vi "Create Pattern Script(Special Frames).vi"(7 "Special Frame Type":T1, 8 "error in (no error)":errorcluster, 10 "Num of Timeset":u32, 11 "BML Pattern Creater in":refnum<class "BML Pattern Creater.lvclass">) -> (0 "error out":errorcluster, 2 "string out":string, 3 "BML Pattern Creater out":refnum<class "BML Pattern Creater.lvclass">)   [LabVIEW 2018, in "BML Pattern Creater.lvlib" / "BML Pattern Creater.lvclass"]
uses:
  BML Pattern Creater.lvclass
  Special Frame.ctl
  Interfaces/Protocol Interface.lvlibp/Interfaces/Protocol Interface/Pin State.ctl
  Interfaces/Protocol Interface.lvlibp/Interfaces/Protocol Interface/Protocol Interface.lvclass
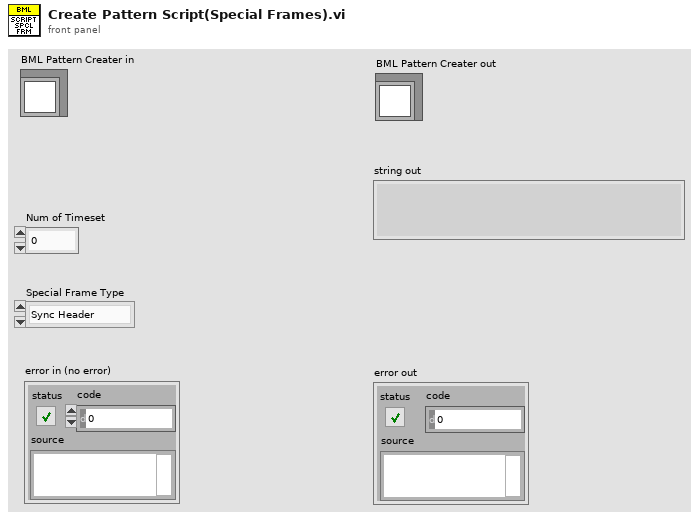
[diagram p1: front panel]
types:
  T1 = typedef "BML Pattern Creater.lvlib/BML Pattern Creater.lvclass/Special Frame.ctl" = enum16{"Sync Header", "BML Header", "SW Trig", "SetID State", "Exit SetID State", "SW Reset", "Wait"}
  T2 = typedef "Protocol Interface.lvlibp/Protocol Interface.lvclass/Pin State.ctl" = enum16{"0", "1", "L", "H", "X", "V", "D", "M"}
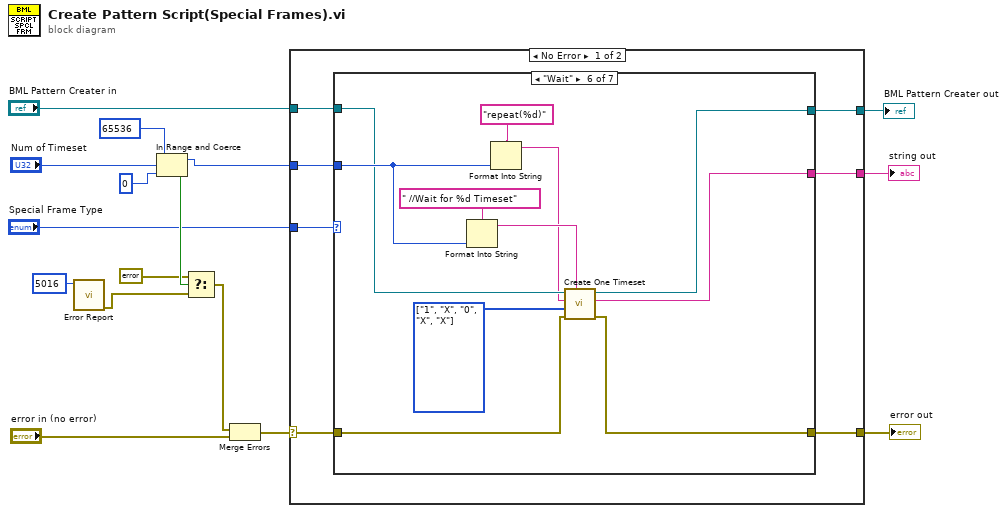
[diagram p0: block diagram]
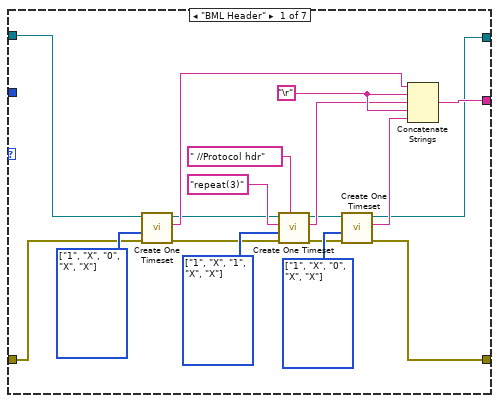
[diagram p2: hidden frame]
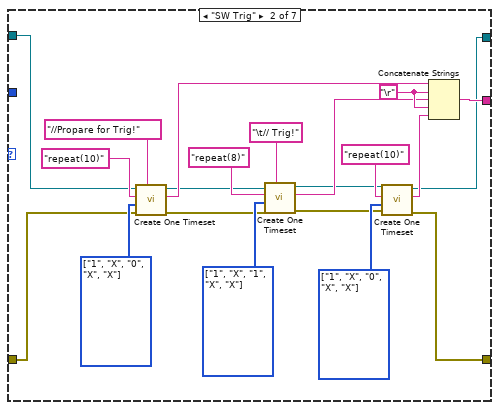
[diagram p3: hidden frame]
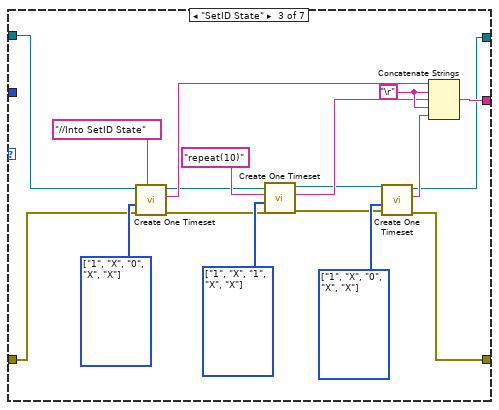
[diagram p4: hidden frame]
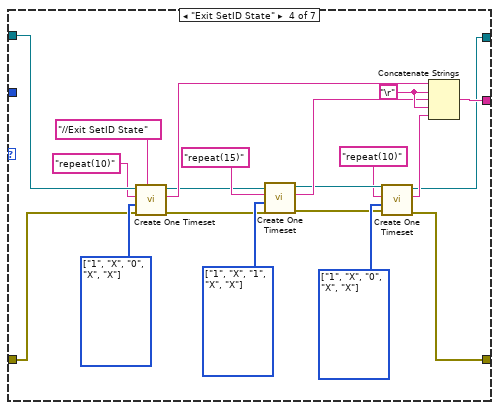
[diagram p5: hidden frame]
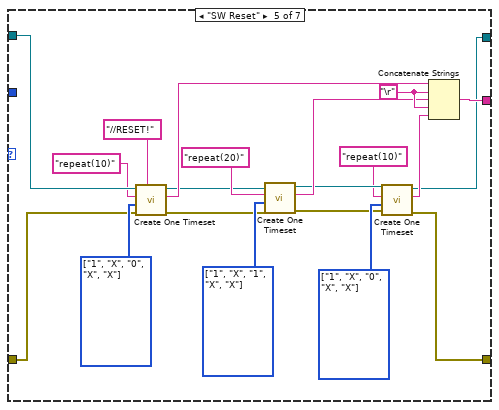
[diagram p6: hidden frame]
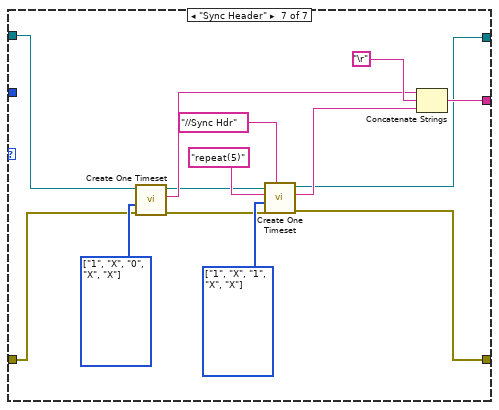
[diagram p7: hidden frame]
diagram:
  n1 = call "Error Report.vi"("Error Code"=i16 5016) -> ("error out"=w7:errorcluster)  [unwired: 10 in]
  n2 = In Range and Coerce(upper limit=u32 65536, x="Num of Timeset", lower limit=u32 0) -> (coerced(x)=w11:u32, In Range?=w10:bool)
  n3 = Select(t=errorcluster {"status"=FALSE, "code"=0, "source"=""} ("error in (no error)"), s=w10, f=w7) -> (s? t:f=w6:errorcluster)
  n4 = Merge Errors(w6, "error in (no error)") -> (w4:errorcluster)
  n5 = case shown="No Error" w4 {
    selector: w4 -> [w20 w147]
    tunnel: [w19 w147] -> w16
    tunnel: "Special Frame Type" -> [w23 _]
    tunnel: [w22 _] -> w15
    tunnel: w11 -> [w21 _]
    tunnel: [w18 w146] -> w2
    tunnel: "BML Pattern Creater in" -> [w17 w146]
    frame No Error {
      n6 = case shown="\"Wait\"" w23 {
        tunnel: [w40 w61 w79 w99 w119 w125 w144] -> w22
        tunnel: w21 -> [_ _ _ _ _ w131 _]
        tunnel: w20 -> [w27 w43 w64 w84 w104 w127 w136]
        tunnel: [w26 w57 w76 w96 w116 w126 w132] -> w19
        tunnel: [w25 w56 w75 w95 w115 w129 w133] -> w18
        tunnel: w17 -> [w24 w42 w63 w83 w103 w128 w135]
        frame "BML Header" {
          w32 = T2[] [enum."1", enum."X", enum."0", enum."X", enum."X"] items=["0", "1", "L", "H", "X", "V", "D", "M"] ("PinState")
          w33 = T2[] [enum."1", enum."X", enum."1", enum."X", enum."X"] items=["0", "1", "L", "H", "X", "V", "D", "M"] ("PinState")
          w34 = T2[] [enum."1", enum."X", enum."0", enum."X", enum."X"] items=["0", "1", "L", "H", "X", "V", "D", "M"] ("PinState")
          w41 = "\r"
          n7 = call-dynamic "Create One Timeset.vi"("error in (no error)"=w27, "Pin State"=w34, "BML Pattern Creater in"=w24) -> ("error out"=w31:errorcluster, "string out"=w39:string, "BML Pattern Creater out"=w28:refnum<class "BML Pattern Creater.lvclass">)  [unwired: 6 in]
          n8 = call-dynamic "Create One Timeset.vi"("Notes"=" //Protocol hdr" ("string"), "error in (no error)"=w31, "Pin State"=w33, "opcode"="repeat(3)", "BML Pattern Creater in"=w28) -> ("error out"=w30:errorcluster, "string out"=w36:string, "BML Pattern Creater out"=w29:refnum<class "BML Pattern Creater.lvclass">)  [unwired: 4 in]
          n9 = call-dynamic "Create One Timeset.vi"("error in (no error)"=w30, "Pin State"=w32, "BML Pattern Creater in"=w29) -> ("error out"=w26:errorcluster, "string out"=w35:string, "BML Pattern Creater out"=w25:refnum<class "BML Pattern Creater.lvclass">)  [unwired: 6 in]
          n10 = Concatenate Strings(w39, w41, w36, w41, w35) -> (w40:string)
        }
        frame "SW Trig" {
          w49 = T2[] [enum."1", enum."X", enum."0", enum."X", enum."X"] items=["0", "1", "L", "H", "X", "V", "D", "M"] ("PinState")
          w52 = T2[] [enum."1", enum."X", enum."1", enum."X", enum."X"] items=["0", "1", "L", "H", "X", "V", "D", "M"] ("PinState")
          w58 = T2[] [enum."1", enum."X", enum."0", enum."X", enum."X"] items=["0", "1", "L", "H", "X", "V", "D", "M"] ("PinState")
          w62 = "\r"
          n11 = call-dynamic "Create One Timeset.vi"("Notes"="//Propare for Trig!", "error in (no error)"=w43, "Pin State"=w49, "opcode"="repeat(10)", "BML Pattern Creater in"=w42) -> ("error out"=w44:errorcluster, "string out"=w46:string, "BML Pattern Creater out"=w45:refnum<class "BML Pattern Creater.lvclass">)  [unwired: 4 in]
          n12 = call-dynamic "Create One Timeset.vi"("Notes"="\t// Trig!", "error in (no error)"=w44, "Pin State"=w52, "opcode"="repeat(8)", "BML Pattern Creater in"=w45) -> ("error out"=w51:errorcluster, "string out"=w55:string, "BML Pattern Creater out"=w50:refnum<class "BML Pattern Creater.lvclass">)  [unwired: 4 in]
          n13 = call-dynamic "Create One Timeset.vi"("error in (no error)"=w51, "Pin State"=w58, "opcode"="repeat(10)", "BML Pattern Creater in"=w50) -> ("error out"=w57:errorcluster, "string out"=w60:string, "BML Pattern Creater out"=w56:refnum<class "BML Pattern Creater.lvclass">)  [unwired: 5 in]
          n14 = Concatenate Strings(w46, w62, w55, w62, w60) -> (w61:string)
        }
        frame "SetID State" {
          w69 = T2[] [enum."1", enum."X", enum."0", enum."X", enum."X"] items=["0", "1", "L", "H", "X", "V", "D", "M"] ("PinState")
          w72 = T2[] [enum."1", enum."X", enum."1", enum."X", enum."X"] items=["0", "1", "L", "H", "X", "V", "D", "M"] ("PinState")
          w77 = T2[] [enum."1", enum."X", enum."0", enum."X", enum."X"] items=["0", "1", "L", "H", "X", "V", "D", "M"] ("PinState")
          w80 = "\r"
          n15 = call-dynamic "Create One Timeset.vi"("Notes"="//Into SetID State", "error in (no error)"=w64, "Pin State"=w69, "BML Pattern Creater in"=w63) -> ("error out"=w65:errorcluster, "string out"=w67:string, "BML Pattern Creater out"=w66:refnum<class "BML Pattern Creater.lvclass">)  [unwired: 5 in]
          n16 = call-dynamic "Create One Timeset.vi"("error in (no error)"=w65, "Pin State"=w72, "opcode"="repeat(10)", "BML Pattern Creater in"=w66) -> ("error out"=w71:errorcluster, "string out"=w74:string, "BML Pattern Creater out"=w70:refnum<class "BML Pattern Creater.lvclass">)  [unwired: 5 in]
          n17 = call-dynamic "Create One Timeset.vi"("error in (no error)"=w71, "Pin State"=w77, "BML Pattern Creater in"=w70) -> ("error out"=w76:errorcluster, "string out"=w78:string, "BML Pattern Creater out"=w75:refnum<class "BML Pattern Creater.lvclass">)  [unwired: 6 in]
          n18 = Concatenate Strings(w67, w80, w74, w80, w78) -> (w79:string)
        }
        frame "Exit SetID State" {
          w89 = T2[] [enum."1", enum."X", enum."0", enum."X", enum."X"] items=["0", "1", "L", "H", "X", "V", "D", "M"] ("PinState")
          w92 = T2[] [enum."1", enum."X", enum."1", enum."X", enum."X"] items=["0", "1", "L", "H", "X", "V", "D", "M"] ("PinState")
          w97 = T2[] [enum."1", enum."X", enum."0", enum."X", enum."X"] items=["0", "1", "L", "H", "X", "V", "D", "M"] ("PinState")
          w100 = "\r"
          n19 = call-dynamic "Create One Timeset.vi"("Notes"="//Exit SetID State", "error in (no error)"=w84, "Pin State"=w89, "opcode"="repeat(10)", "BML Pattern Creater in"=w83) -> ("error out"=w85:errorcluster, "string out"=w87:string, "BML Pattern Creater out"=w86:refnum<class "BML Pattern Creater.lvclass">)  [unwired: 4 in]
          n20 = call-dynamic "Create One Timeset.vi"("error in (no error)"=w85, "Pin State"=w92, "opcode"="repeat(15)", "BML Pattern Creater in"=w86) -> ("error out"=w91:errorcluster, "string out"=w94:string, "BML Pattern Creater out"=w90:refnum<class "BML Pattern Creater.lvclass">)  [unwired: 5 in]
          n21 = call-dynamic "Create One Timeset.vi"("error in (no error)"=w91, "Pin State"=w97, "opcode"="repeat(10)", "BML Pattern Creater in"=w90) -> ("error out"=w96:errorcluster, "string out"=w98:string, "BML Pattern Creater out"=w95:refnum<class "BML Pattern Creater.lvclass">)  [unwired: 5 in]
          n22 = Concatenate Strings(w87, w100, w94, w100, w98) -> (w99:string)
        }
        frame "SW Reset" {
          w109 = T2[] [enum."1", enum."X", enum."0", enum."X", enum."X"] items=["0", "1", "L", "H", "X", "V", "D", "M"] ("PinState")
          w112 = T2[] [enum."1", enum."X", enum."1", enum."X", enum."X"] items=["0", "1", "L", "H", "X", "V", "D", "M"] ("PinState")
          w117 = T2[] [enum."1", enum."X", enum."0", enum."X", enum."X"] items=["0", "1", "L", "H", "X", "V", "D", "M"] ("PinState")
          w120 = "\r"
          n23 = call-dynamic "Create One Timeset.vi"("Notes"="//RESET!", "error in (no error)"=w104, "Pin State"=w109, "opcode"="repeat(10)", "BML Pattern Creater in"=w103) -> ("error out"=w105:errorcluster, "string out"=w107:string, "BML Pattern Creater out"=w106:refnum<class "BML Pattern Creater.lvclass">)  [unwired: 4 in]
          n24 = call-dynamic "Create One Timeset.vi"("error in (no error)"=w105, "Pin State"=w112, "opcode"="repeat(20)", "BML Pattern Creater in"=w106) -> ("error out"=w111:errorcluster, "string out"=w114:string, "BML Pattern Creater out"=w110:refnum<class "BML Pattern Creater.lvclass">)  [unwired: 5 in]
          n25 = call-dynamic "Create One Timeset.vi"("error in (no error)"=w111, "Pin State"=w117, "opcode"="repeat(10)", "BML Pattern Creater in"=w110) -> ("error out"=w116:errorcluster, "string out"=w118:string, "BML Pattern Creater out"=w115:refnum<class "BML Pattern Creater.lvclass">)  [unwired: 5 in]
          n26 = Concatenate Strings(w107, w120, w114, w120, w118) -> (w119:string)
        }
        frame "Wait" {
          w130 = T2[] [enum."1", enum."X", enum."0", enum."X", enum."X"] items=["0", "1", "L", "H", "X", "V", "D", "M"] ("PinState")
          n27 = Format Into String(format string=" //Wait for %d Timeset", w131) -> (resulting string=w123:string)  [unwired: 2 in, 1 out]
          n28 = Format Into String(format string="repeat(%d)", w131) -> (resulting string=w122:string)  [unwired: 2 in, 1 out]
          n29 = call-dynamic "Create One Timeset.vi"("Notes"=w123, "error in (no error)"=w127, "Pin State"=w130, "opcode"=w122, "BML Pattern Creater in"=w128) -> ("error out"=w126:errorcluster, "string out"=w125:string, "BML Pattern Creater out"=w129:refnum<class "BML Pattern Creater.lvclass">)  [unwired: 4 in]
        }
        frame "Sync Header" {
          w140 = T2[] [enum."1", enum."X", enum."0", enum."X", enum."X"] items=["0", "1", "L", "H", "X", "V", "D", "M"] ("PinState")
          w141 = T2[] [enum."1", enum."X", enum."1", enum."X", enum."X"] items=["0", "1", "L", "H", "X", "V", "D", "M"] ("PinState")
          n30 = call-dynamic "Create One Timeset.vi"("error in (no error)"=w136, "Pin State"=w140, "BML Pattern Creater in"=w135) -> ("error out"=w137:errorcluster, "string out"=w139:string, "BML Pattern Creater out"=w138:refnum<class "BML Pattern Creater.lvclass">)  [unwired: 6 in]
          n31 = call-dynamic "Create One Timeset.vi"("Notes"="//Sync Hdr" ("opcode"), "error in (no error)"=w137, "Pin State"=w141, "opcode"="repeat(5)", "BML Pattern Creater in"=w138) -> ("error out"=w132:errorcluster, "string out"=w143:string, "BML Pattern Creater out"=w133:refnum<class "BML Pattern Creater.lvclass">)  [unwired: 4 in]
          n32 = Concatenate Strings(w139, "\r", w143) -> (w144:string)
        }
      }
    }
    frame Error {
    }
  }
  "error out" <- w16
  "string out" <- w15
  "BML Pattern Creater out" <- w2
